vi "Setup VI for Full Screen.vi"(8 "Error In":errorcluster, 11 "This VI":refnum<vi>) -> (0 "Error Out":errorcluster, 3 "VI Ref Out":refnum<vi>)   [LabVIEW 2014]
uses:
  <vilib>/Utility/miscctls.llb/LVPointTypeDef.ctl
  <vilib>/Utility/miscctls.llb/LVRectTypeDef.ctl
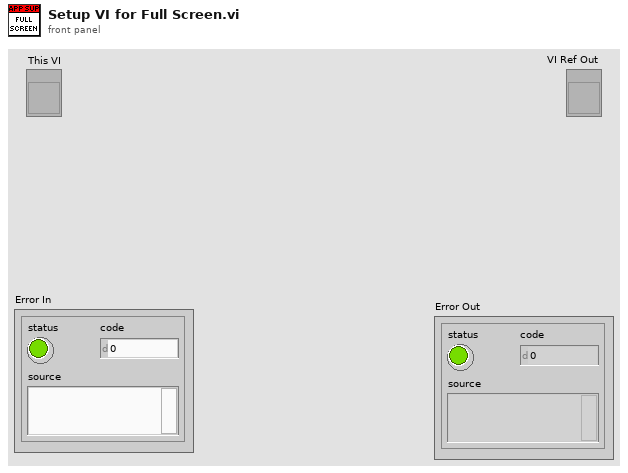
[diagram p1: front panel]
types:
  T1 = typedef "LVRectTypeDef.ctl" = cluster{"Left":i16, "Top":i16, "Right":i16, "Bottom":i16}
  T2 = typedef "LVPointTypeDef.ctl" = cluster{"Horizontal":i16, "Vertical":i16}
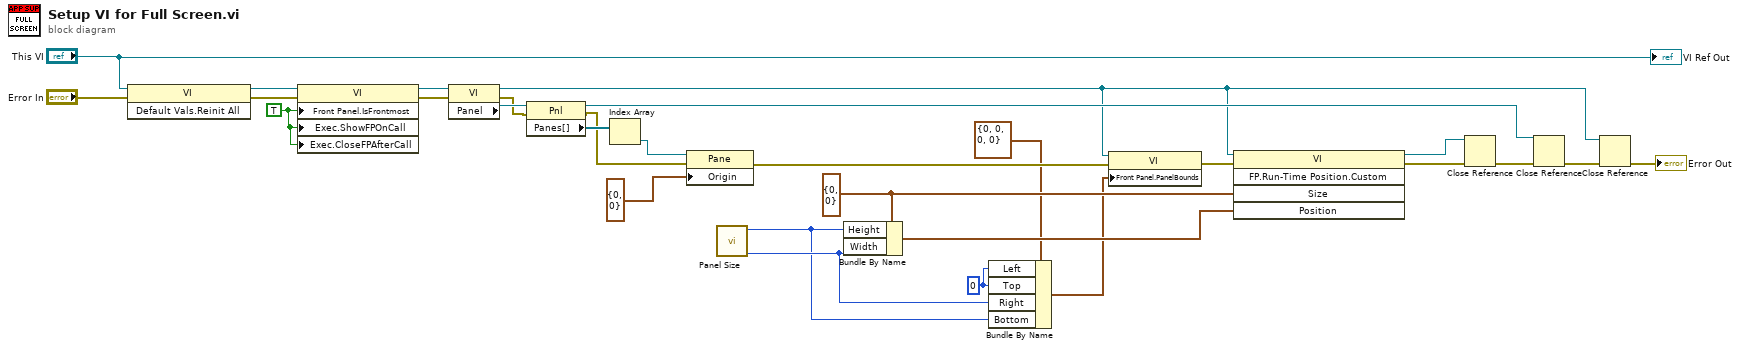
[diagram p0: block diagram]
diagram:
  w2 = i16 0 ("Top")
  w11 = TRUE ("Front Panel Window:Is Frontmost")
  w10 = cluster{"Height":i16, "Width":i16} {"Height"=0, "Width"=0} ("Size")
  n1 = invoke class="VI" method="Default Vals.Reinit All"(reference="This VI", error in="Error In") -> (reference out=w15:refnum<vi>, error out=w12:errorcluster)  [unwired: 1 in, 1 out]
  n2 = property on="Property Node" class="VI"(reference=w15, error in=w12, "Front Panel.IsFrontmost"=w11, "Exec.ShowFPOnCall"=w11, "Exec.CloseFPAfterCall"=w11) -> (reference out=w14:refnum<vi>, error out=w13:errorcluster)
  n3 = property on="Property Node" class="VI"(reference=w14, error in=w13) -> (reference out=w7:refnum<vi>, error out=w21:errorcluster, "Panel"=w25:refnum<vi>)
  n4 = property on="Property Node" class="Pnl"(reference=w25, error in=w21) -> (reference out=w18:refnum<vi>, error out=w20:errorcluster, "Panes[]"=w24:refnum<vi>[])
  n5 = Index Array(array=w24) -> (element=w23:refnum<vi>)  [unwired: 1 in]
  n6 = property on="Property Node" class="Pane"(reference=w23, error in=w20, "Origin"=T2 {"Horizontal"=0, "Vertical"=0}) -> (error out=w8:errorcluster)  [unwired: 1 out]
  n7 = call "Panel Size.vi"() -> ("Width In Pixels"=w4:i32, "Height In pixels"=w3:i32)  [unwired: 10 in]
  n8 = Bundle By Name(cluster=w10, "Height"=w3, "Width"=w4) -> (w6:cluster{"Height":i16, "Width":i16})
  n9 = Bundle By Name(cluster=T1 {"Left"=0, "Top"=0, "Right"=0, "Bottom"=0} ("Front Panel Window:Panel Bounds"), "Left"=w2, "Top"=w2, "Right"=w4, "Bottom"=w3) -> (w1:T1)
  n10 = property class="VI"(reference=w7, error in=w8, "Front Panel.PanelBounds"=w1) -> (error out=w9:errorcluster)  [unwired: 1 out]
  n11 = invoke class="VI" method="FP.Run-Time Position.Custom"(reference=w7, error in=w9, "Size"=w10, "Position"=w6) -> (reference out=w29:refnum<vi>, error out=w28:errorcluster)  [unwired: 1 in, 3 out]
  n12 = Close Reference(reference=w29, error in (no error)=w28) -> (error out=w19:errorcluster)
  n13 = Close Reference(reference=w18, error in (no error)=w19) -> (error out=w17:errorcluster)
  n14 = Close Reference(reference=w7, error in (no error)=w17) -> (error out=→"Error Out":errorcluster)
  "VI Ref Out" <- "This VI"
